vi "SI prefix.vi"(9 "Array":dbl[](array[numeric]), 10 "Numeric":dbl format="%#_8f", 11 "Unit":string) -> (1 "Scaled Array":dbl[](array[numeric]), 2 "Scaled Number":dbl, 3 "modified unit":string)   [LabVIEW 2012, in "Design Server.lvlib"]
uses:
  Design Server.lvlib
panel:
  out "log(x)":dbl
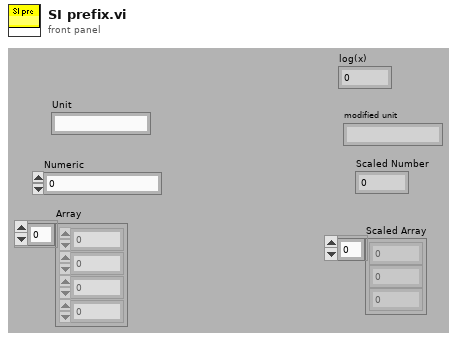
[diagram p1: front panel]
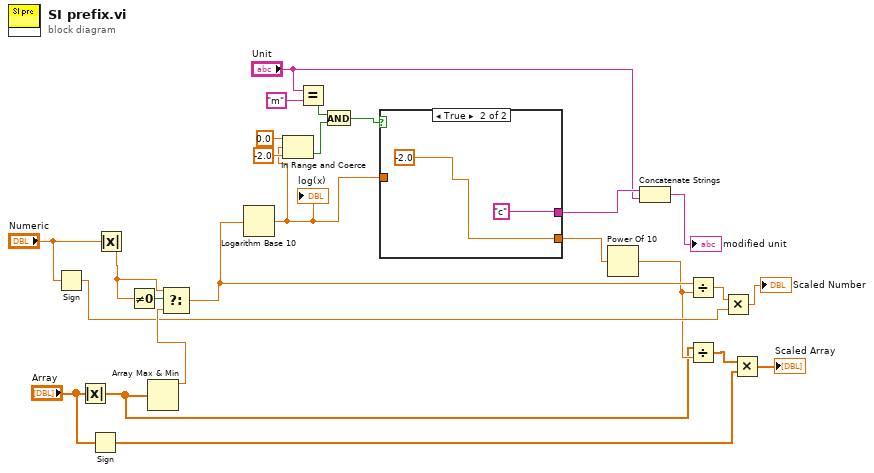
[diagram p0: block diagram]
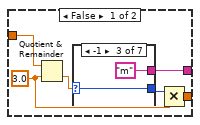
[diagram p2: hidden frame]
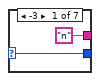
[diagram p3: hidden frame]
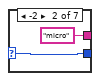
[diagram p4: hidden frame]
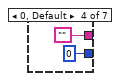
[diagram p5: hidden frame]
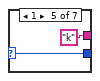
[diagram p6: hidden frame]
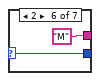
[diagram p7: hidden frame]
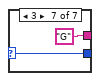
[diagram p8: hidden frame]
diagram:
  n1 = Sign(1:"Numeric") -> (0:w17:dbl)
  n2 = Absolute Value(x="Array") -> (abs(x)=w11:dbl[])
  n3 = Sign(1:"Array") -> (0:w16:dbl[])
  n4 = Absolute Value(x="Numeric") -> (abs(x)=w21:dbl)
  n5 = Not Equal To 0?(x=w21) -> (x != 0?=w24:bool)
  n6 = Array Max & Min(array=w11) -> (max value=w22:dbl)  [unwired: 3 out]
  n7 = Select(t=w21, s=w24, f=w22) -> (s? t:f=w23:dbl)
  n8 = Logarithm Base 10(1:w23) -> (0:w1:dbl)
  "log(x)" <- w1
  n9 = In Range and Coerce(upper limit=0.0, x=w1, lower limit=-2.0) -> (In Range?=w4:bool)  [unwired: 1 out]
  n10 = Equal?(x="Unit", y="m") -> (x = y?=w7:bool)
  n11 = And(x=w7, y=w4) -> (x .and. y?=w3:bool)
  n12 = case shown="True" w3 {
    tunnel: [w31 "c"] -> w25
    tunnel: [w29 -2.0 ("x")] -> w2
    tunnel: w1 -> [w28 _]
    frame False {
      w27 = 3.0 ("y")
      n13 = Quotient & Remainder(x=w28, y=w27) -> (floor(x/y)=w26:dbl)  [unwired: 1 out]
      n14 = case shown="-1" w26 {
        selector: w26 -> [w32 w35 w36 _ w40 w42 w44]
        tunnel: ["n" "micro" "m" "" "k" "M" "G"] -> w31
        tunnel: [w32 w35 w36 0 w40 w42 w44] -> w30
        frame -3 {
        }
        frame -2 {
        }
        frame -1 {
        }
        frame 0, Default {
        }
        frame 1 {
        }
        frame 2 {
        }
        frame 3 {
        }
      }
      n15 = Multiply(x=w30, y=w27) -> (x*y=w29:dbl)
    }
    frame True {
    }
  }
  n16 = Power Of 10(x=w2) -> (10^x=w12:dbl)
  n17 = Concatenate Strings(w25, "Unit") -> (→"modified unit":string)
  n18 = Divide(x=w23, y=w12) -> (x/y=w14:dbl)
  n19 = Divide(x=w11, y=w12) -> (x/y=w13:dbl[])
  n20 = Multiply(x=w14, y=w17) -> (x*y=→"Scaled Number":dbl)
  n21 = Multiply(x=w13, y=w16) -> (x*y=→"Scaled Array":dbl[])
